vi "DistanzaTraParticelle.vi"() -> ()   [LabVIEW 2020]
panel:
  out "Image":T1(plugin-control)
  out "error out":errorcluster
  in  "error in (no error)":errorcluster
  in  "Calibration Image":path=path "C:/Users/Dell/Documents/Sistemi di visione/ProgrammiCompleti/Image/calib-info.png"
  in  "Image Path":path=path "C:/Users/Dell/Documents/Sistemi di visione/ProgrammiCompleti/Image/Piastra.png"
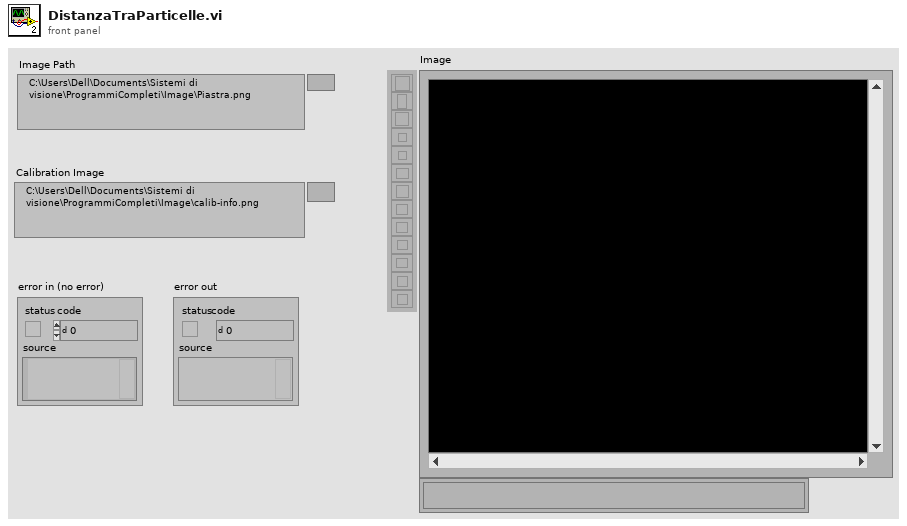
[diagram p1: front panel]
types:
  T1 = typedef "IMAQ Image.ctl" = refnum<image>
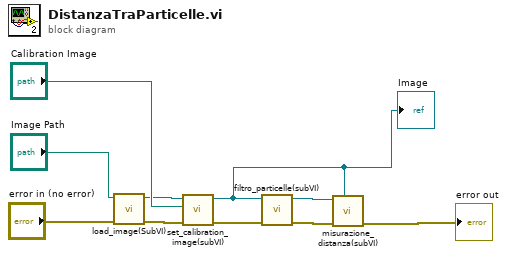
[diagram p0: block diagram]
diagram:
  n1 = call "load_image(SubVI).vi"("error in (no error)"="error in (no error)", "Image Path"="Image Path") -> ("error out"=w6:errorcluster, "Image GRAY"=w2:T1)  [unwired: 8 in]
  n2 = call "set_calibration_image(subVI).vi"("error in (no error)"=w6, "File Path"="Calibration Image", "Image Dst"=w2) -> ("error out"=w5:errorcluster, "Image Out"=w1:T1)  [unwired: 6 in, 1 out]
  "Image" <- w1
  n3 = call "filtro_particelle(subVI).vi"("error in (no error)"=w5, "Image Src"=w1) -> ("error out"=w4:errorcluster, "Image"=w8:T1)  [unwired: 8 in]
  n4 = call "misurazione_distanza(subVI).vi"("Image Dst"=w1, "error in (no error)"=w4, "Image SRC"=w8) -> ("error out"=→"error out":errorcluster)  [unwired: 8 in]
